vi "Get Keys Enumerator.vi"(8 "error in (no error)":errorcluster caption="错误输入（无错误）", 11 "HashTable 输入":refnum<class "HashTable.lvclass"> caption="DNL_LabVIEW Object in") -> (0 "error out":errorcluster caption="错误输出", 2 "Enumerator 输出":refnum<class "Enumerator.lvclass">, 3 "HashTable 输出":refnum<class "HashTable.lvclass"> caption="DNL_LabVIEW Object out")   [LabVIEW 2012, in "HashTable.lvclass"]
uses:
  HashTable.lvclass
  Enumerator/Enumerator.lvclass
  HashTable.lvclass/HashTable.ctl
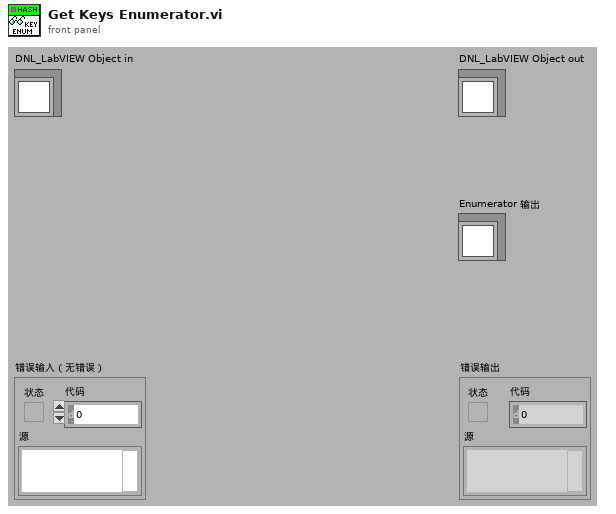
[diagram p1: front panel]
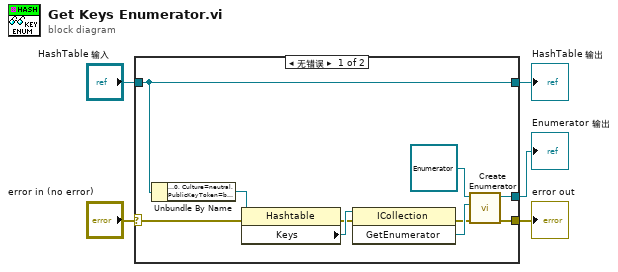
[diagram p0: block diagram]
diagram:
  n1 = case shown="无错误" "error in (no error)" {
    selector: "error in (no error)" -> [w10 w17]
    tunnel: [w6 w17] -> w4
    tunnel: [w15 w16] -> w2
    tunnel: "HashTable 输入" -> [w15 w16]
    tunnel: [w7 _] -> w1
    frame No Error {
      n2 = Unbundle By Name(w15) -> ("HashTable"=w14:refnum<k24>)
      n3 = property class="Hashtable"(reference=w14, error in=w10) -> (error out=w9:errorcluster, "Keys"=w13:refnum<k24>)  [unwired: 1 out]
      n4 = invoke class="ICollection" method="GetEnumerator"(reference=w13, error in=w9) -> (error out=w8:errorcluster, "GetEnumerator"=w12:refnum<k24>)  [unwired: 1 in, 1 out]
      n5 = call "Create Enumerator.vi"("error in (no error)"=w8, "Enumerator"=w12, "Enumerator 输入"=refnum<class "Enumerator.lvclass"> refnum ("Enumerator.lvclass")) -> ("error out"=w6:errorcluster, "Enumerator 输出"=w7:refnum<class "Enumerator.lvclass">)  [unwired: 7 in]
    }
    frame Error {
    }
  }
  "error out" <- w4
  "HashTable 输出" <- w2
  "Enumerator 输出" <- w1
